vi "CarWash_1-AlarmsList.vi"() -> ()   [LabVIEW 2021]
uses:
  Global-Var-OperService.vi
  Global-Var-Simulator.vi
  Global-Var-ControlPanel.vi
panel:
  in  "home_btn":bool
  in  "delete_all_alarams":bool
  out "broken_nozzle":bool
  out "high_temp":bool
  out "high_press":bool
  out "pump_clogged":bool
  out "shiner_low_level":bool
  out "soap_low_level":bool
  out "water_low_level":bool
  # "Niski poziom wody"
  # "Niski poziom mydła"
  # "Niski poziom nabłyszczacza"
  # "Zatkana pompa"
  # "Wysokie ciśnienie"
  # "Wysoka temperatura"
  # "Złamana dysza"
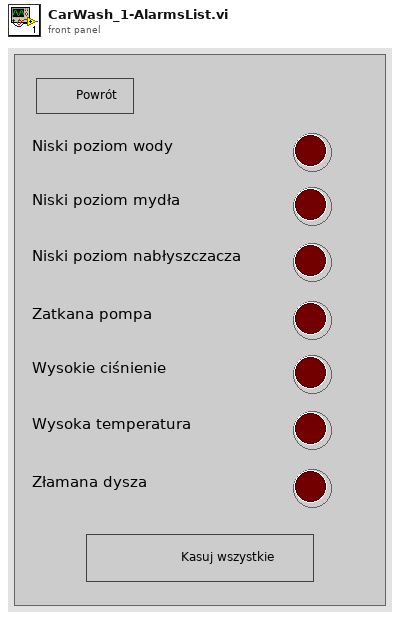
[diagram p1: front panel]
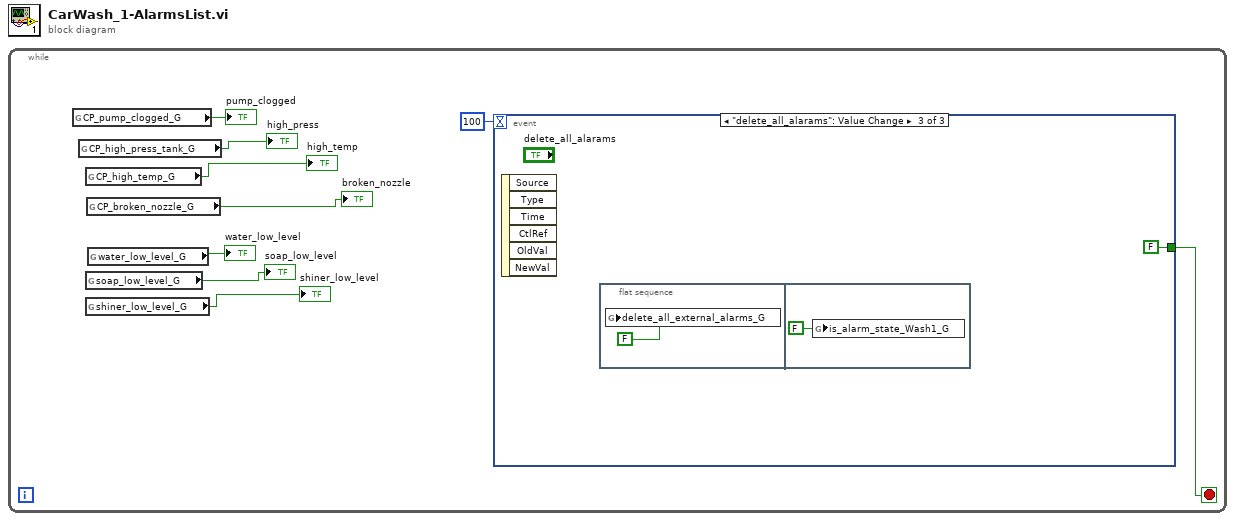
[diagram p0: block diagram]
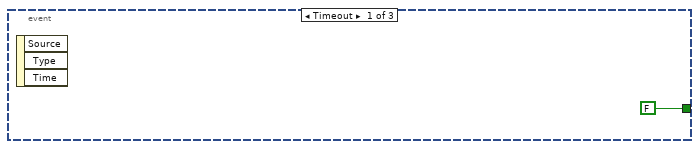
[diagram p2: hidden frame]
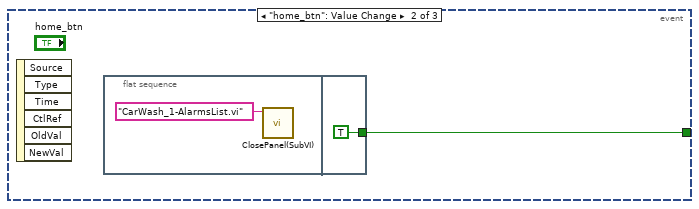
[diagram p3: hidden frame]
diagram:
  n1 = while {
    stop <- w8 stop-if-true
    n2 = global read "Global-Var-ControlPanel.vi" "CP_pump_clogged_G"() -> (→"pump_clogged":bool)
    n3 = global read "Global-Var-ControlPanel.vi" "CP_high_press_tank_G"() -> (→"high_press":bool)
    n4 = global read "Global-Var-ControlPanel.vi" "CP_high_temp_G"() -> (→"high_temp":bool)
    n5 = global read "Global-Var-Simulator.vi" "soap_low_level_G"() -> (→"soap_low_level":bool)
    n6 = global read "Global-Var-Simulator.vi" "shiner_low_level_G"() -> (→"shiner_low_level":bool)
    n7 = global read "Global-Var-ControlPanel.vi" "CP_broken_nozzle_G"() -> (→"broken_nozzle":bool)
    n8 = global read "Global-Var-Simulator.vi" "water_low_level_G"() -> (→"water_low_level":bool)
    n9 = event shown="[2] \"delete_all_alarams\": Value Change" {
      selector: _ -> [_ _ _]
      dyn-events: _ -> [_ _ _]
      timeout: 100 -> [_ _ _]
      tunnel: [FALSE w11 FALSE] -> w8
      event Timeout {
        n10 = event-data() -> ()  [unwired: 1 in, 3 out]
      }
      event "home_btn": Value Change {
        n11 = event-data() -> ()  [unwired: 1 in, 6 out]
        n12 = flat-sequence {
          tunnel: [TRUE] -> w11
          frame #0 {
            n13 = call "ClosePanel(SubVI).vi"("String"="CarWash_1-AlarmsList.vi") -> ()  [unwired: 11 in]
          }
          frame #1 {
          }
        }
      }
      event "delete_all_alarams": Value Change {
        n14 = event-data() -> ()  [unwired: 1 in, 6 out]
        n15 = flat-sequence {
          frame #0 {
            n16 = global write "Global-Var-OperService.vi" "delete_all_external_alarms_G"(FALSE ("service_Sent_G")) -> ()
          }
          frame #1 {
            n17 = global write "Global-Var-Simulator.vi" "is_alarm_state_Wash1_G"(FALSE ("is_alarm_state_Wash1_G")) -> ()
          }
        }
      }
    }
  }
